vi "NI-DMM Specific Logic.vi"(8 "error in":errorcluster, 10 "Measurement Configuration":T1={"pin_name"="", "Range"=10.0, "Measurement Type"=enum."DC Volts", "Resolution in Digits"=5.5} {"Resolution in Digits" items=["3 1/2"=3.5, "4 1/2"=4.5, "5 1/2"=5.5, "6 1/2"=6.5, "7 1/2"=7.5]; "Range" format="%.2f"}, 11 "instrument handle":refnum<k15>) -> (0 "error out":errorcluster, 2 "Measurement Results":T4 {"Absolute Resolution" format="%#_3p"; "Measurement" format="%.6p"}, 3 "instrument handle out":refnum<k15>)   [LabVIEW 2020, in "NIDmmMeasurement.lvlib"]
uses:
  NIDmmMeasurement.lvlib
  Measurement Results.ctl
  Measurement Configuration.ctl
  <instrlib>/niDMM/nidmm.llb/niDMM Function.ctl
  <instrlib>/niDMM/nidmm.llb/niDMM Resolution in Digits.ctl
  <instrlib>/niDMM/nidmm.llb/niDMM Configure Measurement Digits.vi
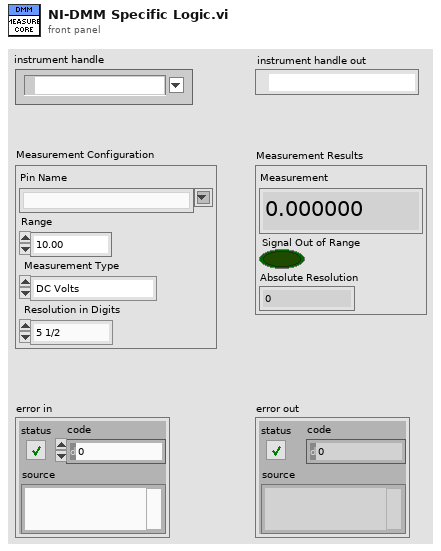
[diagram p1: front panel]
types:
  T1 = typedef "NIDmmMeasurement.lvlib/Measurement Configuration.ctl" = cluster{"pin_name":string, "Range":dbl, "Measurement Type":T2, "Resolution in Digits":T3}
  T2 = typedef "niDMM Function.ctl" = enum16{"DC Volts", "AC Volts", "DC Current", "AC Current", "2-wire Resistance", "4-wire Resistance", "Diode", "Frequency", "Period", "AC Volts DC Coupled", "Capacitance", "Inductance", "Temperature"}
  T3 = typedef "niDMM Resolution in Digits.ctl" = dbl
  T4 = typedef "NIDmmMeasurement.lvlib/Measurement Results.ctl" = cluster{"Measurement ":dbl, "Signal Out of Range":bool, "Absolute Resolution":dbl}
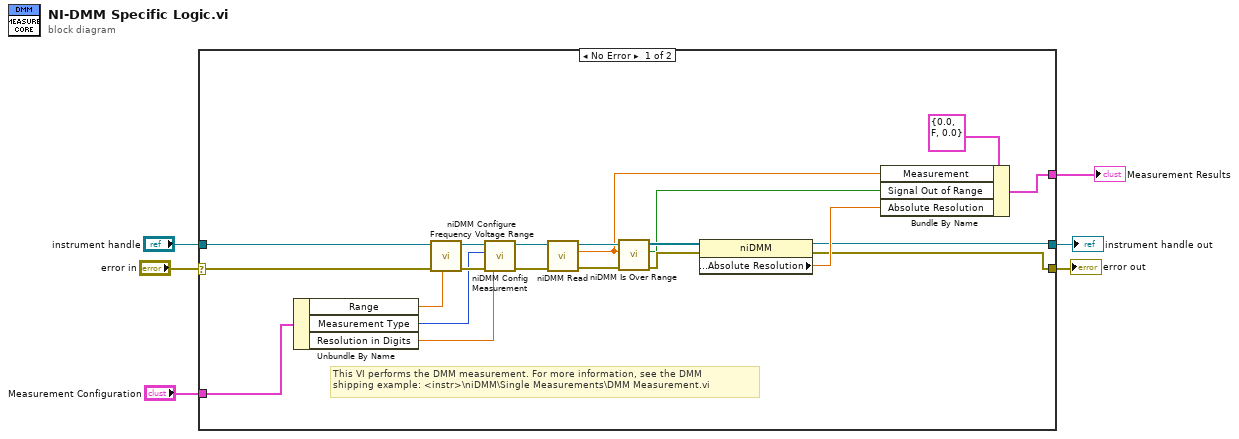
[diagram p0: block diagram]
diagram:
  n1 = case shown="No Error" "error in" {
    selector: "error in" -> [w7 w28]
    tunnel: "Measurement Configuration" -> [w27 _]
    tunnel: [w26 _] -> w2
    tunnel: [w11 w28] -> w6
    tunnel: "instrument handle" -> [w8 w29]
    tunnel: [w12 w29] -> w3
    frame No Error {
      # "This VI performs the DMM measurement. For more information, see the DMM\nshipping example: <instr>\\niDMM\\Single Measurements\\DMM Measurement.vi"
      n2 = Unbundle By Name(w27) -> ("Range"=w10:dbl, "Measurement Type"=w18:T2, "Resolution in Digits"=w21:T3)
      n3 = call <instrlib>:"niDMM Configure Frequency Voltage Range.vi"("Frequency Voltage Range"=w10, "error in (no error)"=w7, "instrument handle"=w8) -> ("error out"=w19:errorcluster, "instrument handle out"=w20:refnum<k15>)  [unwired: 7 in]
      n4 = call-poly <instrlib>:"niDMM Config Measurement.vi"("Range"=w21, "error in (no error)"=w19, "Function"=w18, "instrument handle"=w20) -> ("error out"=w25:errorcluster, "instrument handle out"=w24:refnum<k15>)  [unwired: 6 in]
      n5 = call <instrlib>:"niDMM Read.vi"("error in (no error)"=w25, "instrument handle"=w24) -> ("error out"=w16:errorcluster, "Measurement"=w13:dbl, "instrument handle out"=w23:refnum<k15>)  [unwired: 7 in]
      n6 = call <instrlib>:"niDMM Is Over Range.vi"("error in (no error)"=w16, "Measurement"=w13, "instrument handle"=w23) -> ("error out"=w17:errorcluster, "Over Range?"=w14:bool, "instrument handle out"=w22:refnum<k15>)  [unwired: 6 in]
      n7 = property class="niDMM"(reference=w22, error in=w17) -> (reference out=w12:refnum<k15>, error out=w11:errorcluster, "Configuration:Absolute Resolution"=w15:dbl)
      n8 = Bundle By Name(cluster=T4 {"Measurement "=0.0, "Signal Out of Range"=FALSE, "Absolute Resolution"=0.0} ("Measurement Results"), "Measurement"=w13, "Signal Out of Range"=w14, "Absolute Resolution"=w15) -> (w26:T4)
    }
    frame Error {
    }
  }
  "error out" <- w6
  "instrument handle out" <- w3
  "Measurement Results" <- w2
